vi "STEPFLAG.vi"(0 "VISA resource name":refnum<visa-resource-name>, 5 "error in (no error)":errorcluster) -> (14 "VISA resource name out":refnum<visa-resource-name>, 15 "Test Step Status Flag":string="\r\n", 16 "Test Step Status Description":string, 17 "Error Message":string, 18 "Error Code":i32, 19 "error out":errorcluster)   [LabVIEW 2010, in "VITREK V7X.lvlib"]
doc: "Responds with a <NR1> indicating the overall test sequence fail status and reason. This is the logical OR of all individual step status flags. This can also be used while running a test sequence.\n\n<b>Note:</b> please refer to the instrument manual for the <b>RSLT?</b> specification (refer to </b>Test Step Status Flags</b> table)."
uses:
  VITREK V7X.lvlib
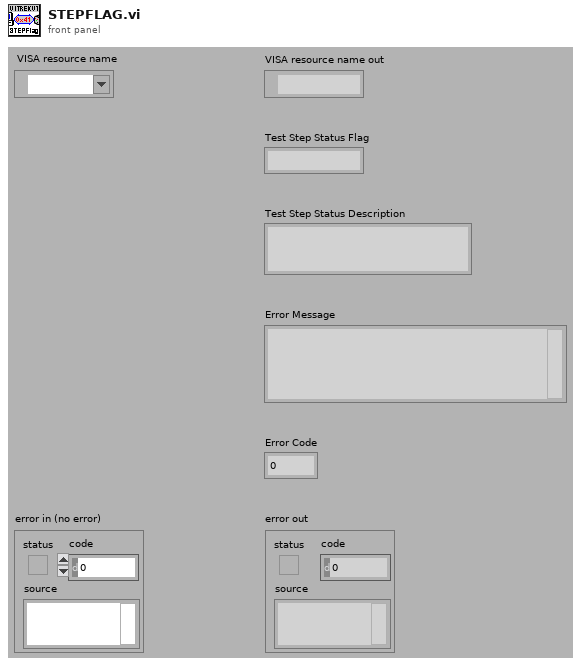
[diagram p1: front panel]
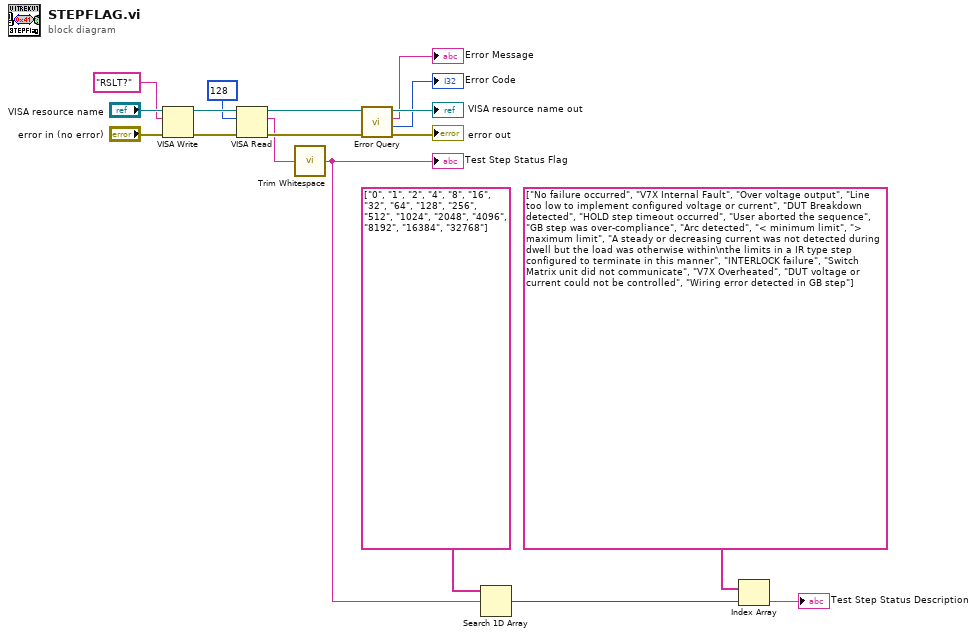
[diagram p0: block diagram]
diagram:
  n1 = VISA Write(VISA resource name="VISA resource name", write buffer="RSLT?", error in (no error)="error in (no error)") -> (VISA resource name out=w14:refnum<visa-resource-name>, error out=w12:errorcluster)  [unwired: 1 out]
  n2 = VISA Read(VISA resource name=w14, byte count=u32 128, error in (no error)=w12) -> (VISA resource name out=w13:refnum<visa-resource-name>, read buffer=w8:string, error out=w9:errorcluster)  [unwired: 1 out]
  n3 = call <vilib>:"Trim Whitespace.vi"("string"=w8) -> ("trimmed string"=w7:string)  [unwired: 1 in]
  "Test Step Status Flag" <- w7
  n4 = call "Error Query.vi"("error in (no error)"=w9, "VISA resource name"=w13) -> ("error out"=→"error out":errorcluster, "Error Code"=→"Error Code":i32, "Error Message"=→"Error Message":string, "VISA resource name out"=→"VISA resource name out":refnum<visa-resource-name>)  [unwired: 6 in]
  n5 = Search 1D Array(1D array=string[] ["0", "1", "2", "4", "8", "16", "32", "64", "128", "256", "512", "1024", "2048", "4096", "8192", "16384", "32768"], element=w7) -> (index of element=w4:i32)  [unwired: 1 in]
  n6 = Index Array(array=string[] ["No failure occurred", "V7X Internal Fault", "Over voltage output", "Line too low to implement configured voltage or current", "DUT Breakdown detected", "HOLD step timeout occurred", "User aborted the sequence", "GB step was over-compliance", "Arc detected", "< minimum limit", "> maximum limit", "A steady or decreasing current was not detected during dwell but the load was otherwise within\nthe limits in a IR type step configured to terminate in this manner", "INTERLOCK failure", "Switch Matrix unit did not communicate", "V7X Overheated", "DUT voltage or current could not be controlled", "Wiring error detected in GB step"], index=w4) -> (element=→"Test Step Status Description":string)
